vi "DEMO.vi"() -> ()   [LabVIEW 2012, in "GZip.lvlib"]
uses:
  GZip.lvlib
panel:
  out "错误输出":errorcluster
  out "DeCompressed String":string
  in  "String":string
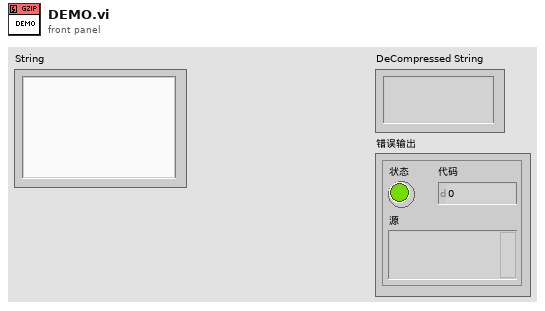
[diagram p1: front panel]
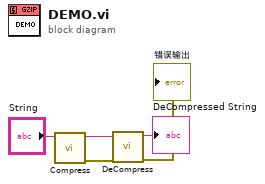
[diagram p0: block diagram]
diagram:
  n1 = call "Compress.vi"("String"="String") -> ("错误输出"=w3:errorcluster, "Compressed String"=w4:string)  [unwired: 8 in, 1 out]
  n2 = call "DeCompress.vi"("错误输入"=w3, "Compressed String"=w4) -> ("错误输出"=→"错误输出":errorcluster, "DeCompressed String"=→"DeCompressed String":string)  [unwired: 8 in]
